vi "GetPosition.vi"(8 "error in":errorcluster, 10 "Channel":u8, 11 "VISA resource name":refnum<visa-resource-name>) -> (0 "error out":errorcluster, 2 "Position":u16, 3 "VISA resource name out":refnum<visa-resource-name>)   [LabVIEW 2023, in "Maestro.lvlib"]
uses:
  Maestro.lvlib
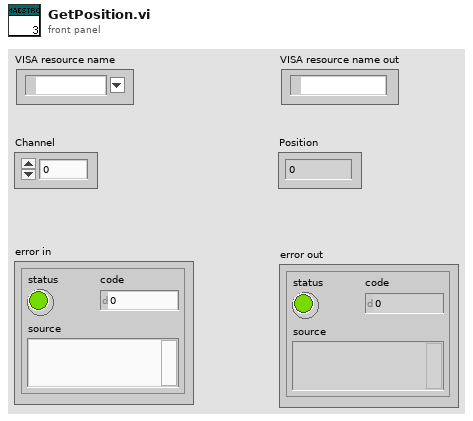
[diagram p1: front panel]
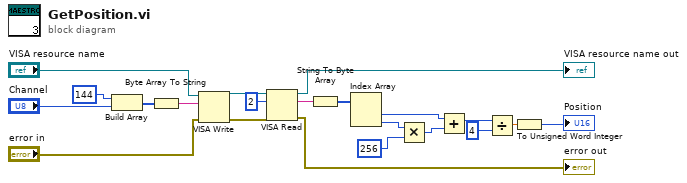
[diagram p0: block diagram]
diagram:
  n1 = Build Array(u8 144, "Channel") -> (w20:u8[])
  n2 = Byte Array To String(unsigned byte array=w20) -> (string=w19:string)
  n3 = VISA Write(VISA resource name="VISA resource name", write buffer=w19, error in (no error)="error in") -> (VISA resource name out=w15:refnum<visa-resource-name>, error out=w14:errorcluster)  [unwired: 1 out]
  n4 = VISA Read(VISA resource name=w15, byte count=u32 2, error in (no error)=w14) -> (VISA resource name out=→"VISA resource name out":refnum<visa-resource-name>, read buffer=w12:string, error out=→"error out":errorcluster)  [unwired: 1 out]
  n5 = String To Byte Array(string=w12) -> (unsigned byte array=w11:u8[])
  n6 = Index Array(array=w11) -> (element #1=w8:u8, element #2=w10:u8)  [unwired: 2 in]
  n7 = Multiply(x=w10, y=u16 256) -> (x*y=w7:u16)
  n8 = Add(x=w8, y=w7) -> (x+y=w4:u16)
  n9 = Divide(x=w4, y=u16 4) -> (x/y=w2:dbl)
  n10 = To Unsigned Word Integer(number=w2) -> (unsigned 16bit integer=→"Position":u16)
